vi "Page Reference.vi"(8 "error in (no error)":errorcluster, 9 "Operation":enum16{"Get", "Set"}(ring), 11 "VI Refnum":refnum<vi>) -> (0 "error out":errorcluster, 3 "VI Refnum (out)":refnum<vi>)   [LabVIEW 2017, in "WebServiceImporter.lvlib" / "Main Panel.lvlib" / "Input Info.lvlib"]
uses:
  <vilib>/Platform/WebService/Main Panel/Pages/Input Info/Input Info.lvlib
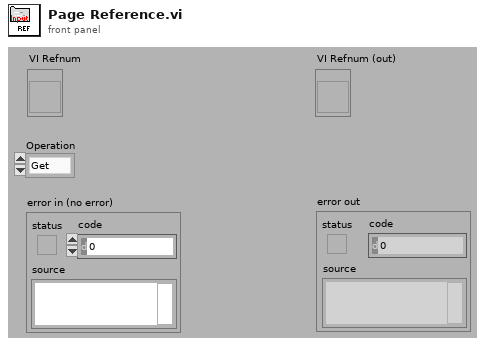
[diagram p1: front panel]
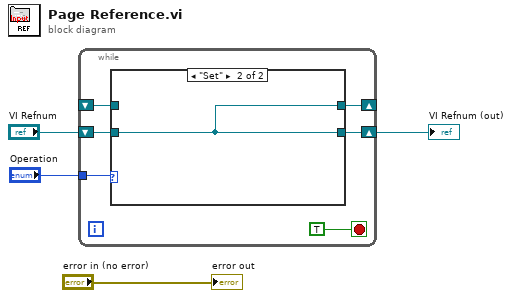
[diagram p0: block diagram]
diagram:
  n1 = while {
    tunnel: "Operation" -> [w9]
    shift-right: [w7] -> w2
    shift-left: "VI Refnum" -> [w8]
    shift-right: [w6] -> _
    shift-left: _ -> [w5]
    stop <- TRUE stop-if-true
    n2 = case shown="\"Set\"" w9 {
      tunnel: w8 -> [_ w12]
      tunnel: [w11 w12] -> w7
      tunnel: [w11 w12] -> w6
      tunnel: w5 -> [w11 _]
      frame "Get", Default {
      }
      frame "Set" {
      }
    }
  }
  "VI Refnum (out)" <- w2
  "error out" <- "error in (no error)"
